vi "Decode JSON List Of Devices.vi"(8 "error in":errorcluster, 11 "table of devices":string[](array[string])) -> (0 "error out":errorcluster, 1 "description of device":string, 2 "name of device":string, 3 "device index":i32)   [LabVIEW 2023, in "DeviceManager.lvlib"]
uses:
  DeviceManager.lvlib
panel:
  # "Connector Pane"
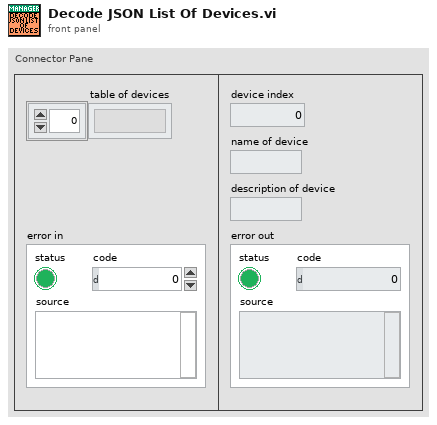
[diagram p1: front panel]
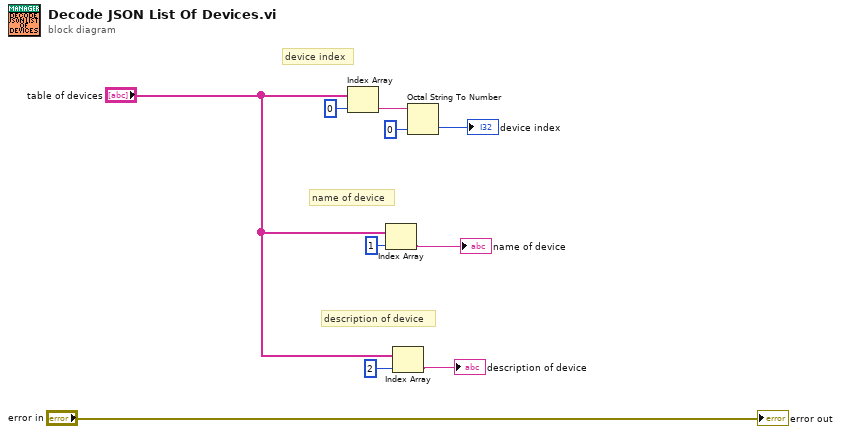
[diagram p0: block diagram]
diagram:
  # "description of device"
  # "name of device"
  # "device index"
  n1 = Index Array(array="table of devices", index=0) -> (element=w6:string)
  n2 = Index Array(array="table of devices", index=1) -> (element=→"name of device":string)
  n3 = Index Array(array="table of devices", index=2) -> (element=→"description of device":string)
  n4 = Octal String To Number(2:0 ("index"), 4:w6) -> (0:→"device index":i32)  [unwired: 1 in, 1 out]
  "error out" <- "error in"
